vi "BRig_RT__Case_Exp__State_Selection__v2.vi"(0 "input_state":T1, 2 "input_dataCurrent":u16[](array[numeric]), 3 "input_dataTrial":u16[][](array[numeric]), 4 "input_dataExp":u16[](array[numeric]), 5 "input_arrTrig":bool[](array[boolean]), 6 "input_SelectWrong":bool, 8 "input_SelectReward":bool, 10 "input_LickR":bool, 12 "input_LickL":bool) -> (7 "output_l2_laserOn":bool, 9 "output_l2_laserEvent":bool, 11 "output_l1_laserOn":bool, 13 "output_l1_laserEvent":bool, 14 "output_state":T1, 16 "output_dataCurrent":u16[](array[numeric]), 17 "output_dataTrial":u16[][](array[numeric]), 18 "output_allReward_L":bool, 19 "output_allReward_R":bool)   [LabVIEW 2014]
uses:
  myRIO_BRig_RT__Case_Exp_stateList.ctl
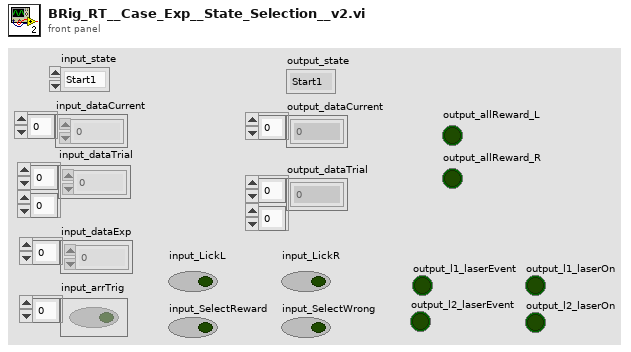
[diagram p1: front panel]
types:
  T1 = typedef "myRIO_BRig_RT__Case_Exp_stateList.ctl" = enum16{"Start1", "Start2", "Start3", "saveSettings1", "saveSettings2", "saveSettings3", "saveSettings4", "saveSettings_LC_ENL_l1", "saveSettings_LC_ENL_l2", "saveSettings_LC_Cue_l1", "saveSettings_LC_Cue_l2", "saveSettings6_LC_l1_Other", "SaveSettings6_LC_l2_Other", "setSettings_Audio", "setSettings_Laser", "initBlock_pre", "initBlock", "initBlock2", "initBlock_post", "initTrial_pre", "initTrial", "initTrial2", "initTrial3", "initTrial4", "initTrial_LC_ENL1", "initTrial_LC_Cue1", "initTrial_LC_Cue1_2", "initTrial_LC_Sel", "initTrial_post", "ENL1_pre", "ENL1", "ENL1_post", "ENL1Penalty_pre", "ENL1Penalty", "ENL2_pre", "ENL2", "ENL2Penalty_pre", "ENL2Penalty", "Cue1_pre", "Cue1", "Cue1_post", "Cue1Penalty_pre", "Cue1Penalty", "Cue2_pre", "Cue2", "Cue2Penalty_pre", "Cue2Penalty", "Selection_pre", "Selection", "Select_post", "SelectReward_pre", "SelectReward", "SelectRewardPost_pre", "SelectRewardPost", "SelectWrong_pre", "SelectWrong", "SelectWrong_post", "SelectTimeout_pre", "SelectTimeout", "SelectTimeout_post", "endTrial_pre", "endTrial1", "endTrial2", "endTrial3", "endTrial_post", "endBlock_pre", "endBlock", "endBlock_post", "endExp", "commConnect", "commUpload_pre", "commUpload_dataBlock", "commUpload_dataCurrent", "commUpload_dataExp", "commUpload_dataLC", "commUpload_dataTrial", "commUpload_post", "saveData_pre", "saveData_dataBlock", "saveData_dataCurrent", "saveData_dataExp", "saveData_dataLC", "saveData_dataTrial", "saveData_post", "empty_endBlock1", "empty_endBlock2", "empty_endTrial1", "empty_endTrial2", "empty_endTrial3", "empty_endTrial4", "empty_endTrial5", "dummyState", "dummyState_endBlock", "FreeReward_pre", "FreeReward", "FreeRewardPost_pre", "FreeRewardPost"}
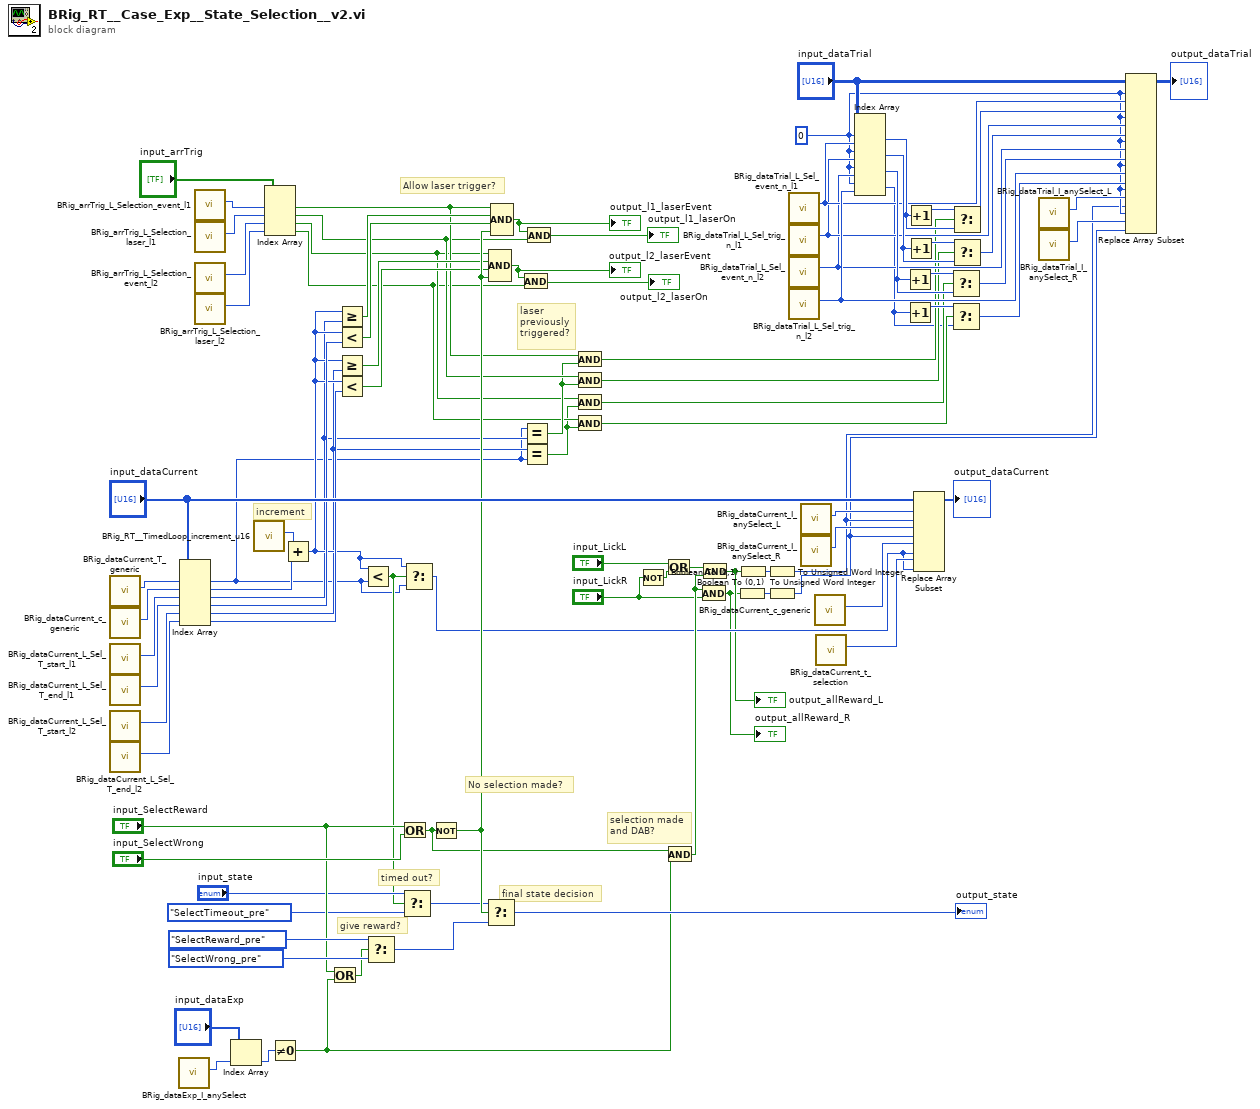
[diagram p0: block diagram]
diagram:
  w12 = 0
  # "laser\npreviously\ntriggered?"
  # "selection made\nand DAB?"
  # "final state decision"
  # "give reward?"
  # "timed out?"
  # "increment"
  # "No selection made?"
  # "Allow laser trigger?"
  n1 = call "BRig_dataCurrent_T_generic.vi"() -> ("output_T_generic"=w55:i32)  [unwired: 11 in]
  n2 = call "BRig_dataCurrent_c_generic.vi"() -> ("output_count_generic"=w54:i32)  [unwired: 11 in]
  n3 = call "BRig_dataCurrent_L_Sel_T_start_l1.vi"() -> ("output_L_Sel_T_start_l1"=w59:i32)  [unwired: 11 in]
  n4 = call "BRig_dataCurrent_L_Sel_T_end_l1.vi"() -> ("output_L_Sel_T_end_l1"=w58:i32)  [unwired: 11 in]
  n5 = call "BRig_dataCurrent_L_Sel_T_start_l2.vi"() -> ("output_L_Sel_T_start_l2"=w57:i32)  [unwired: 11 in]
  n6 = call "BRig_dataCurrent_L_Sel_T_end_l2.vi"() -> ("output_L_Sel_T_end_l2"=w56:i32)  [unwired: 11 in]
  n7 = call "BRig_dataExp_I_anySelect.vi"() -> ("output_I_anySelect"=w85:i32)  [unwired: 11 in]
  n8 = Index Array(array="input_dataCurrent", index #1=w55, index #2=w54, index #3=w59, index #4=w58, index #5=w57, index #6=w56) -> (element #1=w38:u16, element #2=w41:u16, element #3=w39:u16, element #4=w52:u16, element #5=w40:u16, element #6=w51:u16)
  n9 = call "BRig_arrTrig_L_Selection_event_l1.vi"() -> ("output_L_Sel_event_l1"=w74:i32)  [unwired: 11 in]
  n10 = call "BRig_arrTrig_L_Selection_laser_l1.vi"() -> ("output_L_Sel_laserTrig_l1"=w73:i32)  [unwired: 11 in]
  n11 = call "BRig_arrTrig_L_Selection_event_l2.vi"() -> ("output_L_Sel_event_l2"=w72:i32)  [unwired: 11 in]
  n12 = call "BRig_arrTrig_L_Selection_laser_l2.vi"() -> ("output_L_Sel_laserTrig_l2"=w71:i32)  [unwired: 11 in]
  n13 = Index Array(array="input_dataExp", index=w85) -> (element=w84:u16)
  n14 = call "BRig_RT__TimedLoop_increment_u16.vi"() -> ("output_increment__u16"=w53:u16)  [unwired: 11 in]
  n15 = Index Array(array="input_arrTrig", index #1=w74, index #2=w73, index #3=w72, index #4=w71) -> (element #1=w37:bool, element #2=w36:bool, element #3=w34:bool, element #4=w33:bool)
  n16 = Not Equal To 0?(x=w84) -> (x != 0?=w60:bool)
  n17 = Add(x=w53, y=w41) -> (x+y=w46:u16)
  n18 = Or(x="input_SelectReward", y=w60) -> (x .or. y?=w63:bool)
  n19 = Greater Or Equal?(x=w46, y=w39) -> (x >= y?=w50:bool)
  n20 = Less?(x=w46, y=w52) -> (x < y?=w49:bool)
  n21 = Greater Or Equal?(x=w46, y=w40) -> (x >= y?=w48:bool)
  n22 = Less?(x=w46, y=w51) -> (x < y?=w47:bool)
  n23 = Less?(x=w46, y=w38) -> (x < y?=w43:bool)
  n24 = Select(t=myRIO_BRig_RT__Case_Exp_stateList."SelectReward_pre" ("Enum"), s=w63, f=myRIO_BRig_RT__Case_Exp_stateList."SelectWrong_pre" ("Enum")) -> (s? t:f=w66:T1)
  n25 = Or(x="input_SelectReward", y="input_SelectWrong") -> (x .or. y?=w61:bool)
  n26 = Select(t="input_state", s=w43, f=myRIO_BRig_RT__Case_Exp_stateList."SelectTimeout_pre" ("Enum")) -> (s? t:f=w42:T1)
  n27 = Select(t=w46, s=w43, f=w38) -> (s? t:f=w3:u16)
  n28 = Not(x=w61) -> (.not. x?=w65:bool)
  n29 = Select(t=w42, s=w65, f=w66) -> (s? t:f=→"output_state":T1)
  n30 = Compound Arithmetic op=AND(w34, w48, w47, w65) -> (w70:bool)
  "output_l2_laserEvent" <- w70
  n31 = Compound Arithmetic op=AND(w37, w50, w49, w65) -> (w69:bool)
  "output_l1_laserEvent" <- w69
  n32 = And(x=w70, y=w33) -> (x .and. y?=→"output_l2_laserOn":bool)
  n33 = Equal?(x=w38, y=w39) -> (x = y?=w35:bool)
  n34 = Equal?(x=w40, y=w38) -> (x = y?=w32:bool)
  n35 = And(x=w69, y=w36) -> (x .and. y?=→"output_l1_laserOn":bool)
  n36 = And(x=w37, y=w35) -> (x .and. y?=w11:bool)
  n37 = And(x=w36, y=w35) -> (x .and. y?=w10:bool)
  n38 = And(x=w34, y=w32) -> (x .and. y?=w9:bool)
  n39 = And(x=w33, y=w32) -> (x .and. y?=w8:bool)
  n40 = Not(x="input_LickR") -> (.not. x?=w76:bool)
  n41 = Or(x="input_LickL", y=w76) -> (x .or. y?=w75:bool)
  n42 = And(x=w61, y=w60) -> (x .and. y?=w81:bool)
  n43 = And(x=w81, y="input_LickR") -> (x .and. y?=w1:bool)
  "output_allReward_R" <- w1
  n44 = And(x=w75, y=w81) -> (x .and. y?=w2:bool)
  "output_allReward_L" <- w2
  n45 = Boolean To (0,1)(Boolean=w1) -> (0, 1=w79:i16)
  n46 = Boolean To (0,1)(Boolean=w2) -> (0, 1=w80:i16)
  n47 = To Unsigned Word Integer(number=w80) -> (unsigned 16bit integer=w6:u16)
  n48 = To Unsigned Word Integer(number=w79) -> (unsigned 16bit integer=w5:u16)
  n49 = call "BRig_dataTrial_L_Sel_event_n_l1.vi"() -> ("output_L_Sel_event_n_l1"=w17:i32)  [unwired: 11 in]
  n50 = call "BRig_dataTrial_L_Sel_trig_n_l1.vi"() -> ("output_L_Sel_trig_n_l1"=w16:i32)  [unwired: 11 in]
  n51 = call "BRig_dataTrial_L_Sel_event_n_l2.vi"() -> ("output_L_Sel_event_n_l2"=w15:i32)  [unwired: 11 in]
  n52 = call "BRig_dataTrial_L_Sel_trig_n_l2.vi"() -> ("output_L_Sel_trig_n_l2"=w18:i32)  [unwired: 11 in]
  n53 = call "BRig_dataCurrent_I_anySelect_L.vi"() -> ("output_IanySelect_L"=w83:i32)  [unwired: 11 in]
  n54 = call "BRig_dataCurrent_I_anySelect_R.vi"() -> ("output_IanySelect_R"=w82:i32)  [unwired: 11 in]
  n55 = call "BRig_dataCurrent_c_generic.vi"() -> ("output_count_generic"=w92:i32)  [unwired: 11 in]
  n56 = call "BRig_dataCurrent_t_selection.vi"() -> ("output_t_selection"=w4:i32)  [unwired: 11 in]
  n57 = Index Array(array="input_dataTrial", index (row) #1=w12, index (col) #1=w17, index (row) #2=w12, index (col) #2=w16, index (row) #3=w12, index (col) #3=w15, index (row) #4=w12, index (col) #4=w18) -> (element #1=w29:u16, element #2=w25:u16, element #3=w24:u16, element #4=w7:u16)
  n58 = Increment(x=w24) -> (x+1=w27:u16)
  n59 = Increment(x=w7) -> (x+1=w26:u16)
  n60 = Increment(x=w29) -> (x+1=w30:u16)
  n61 = Increment(x=w25) -> (x+1=w28:u16)
  n62 = Replace Array Subset(array="input_dataCurrent", new element #1=w6, index #1=w83, new element #2=w5, index #2=w82, new element #3=w3, index #3=w92, new element #4=w3, index #4=w4) -> (→"output_dataCurrent":u16[])
  n63 = Select(t=w27, s=w9, f=w24) -> (s? t:f=w21:u16)
  n64 = Select(t=w26, s=w8, f=w7) -> (s? t:f=w20:u16)
  n65 = Select(t=w30, s=w11, f=w29) -> (s? t:f=w23:u16)
  n66 = Select(t=w28, s=w10, f=w25) -> (s? t:f=w22:u16)
  n67 = call "BRig_dataTrial_I_anySelect_L.vi"() -> ("output_I_allReward_L"=w14:i32)  [unwired: 11 in]
  n68 = call "BRig_dataTrial_I_anySelect_R.vi"() -> ("output_I_anySelect_R"=w13:i32)  [unwired: 11 in]
  n69 = Replace Array Subset(array="input_dataTrial", new element #1=w23, index (row) #1=w12, index (col) #1=w17, new element #2=w22, index (row) #2=w12, index (col) #2=w16, new element #3=w21, index (row) #3=w12, index (col) #3=w15, new element #4=w20, index (row) #4=w12, index (col) #4=w18, new element #5=w6, index (row) #5=w12, index (col) #5=w14, new element #6=w5, index (row) #6=w12, index (col) #6=w13) -> (→"output_dataTrial":u16[][])
